vi "go striaght.vi"(7 "距离":i32, 8 "error in (no error)":errorcluster, 11 "KNR in":T1) -> (0 "error out":errorcluster, 3 "KNR out":T1)   [LabVIEW 2013]
uses:
  <userlib>/KNR OS 3.0 LabVIEW Toolkit/Type Definition/KNR3 Reference.ctl
  <userlib>/_FPGA Interface Advanced Tools/FPGA Interface Base/FPGA Interface Base.lvclass
  <userlib>/KNR OS 3.0 LabVIEW Toolkit/Type Definition/Resource.ctl
  Global 1.vi
panel:
  out "右轮位置":i32
  out "右轮初始位置":i32
  out "右轮移动了":i32
  in  "STOP":bool
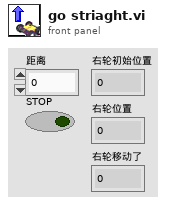
[diagram p1: front panel]
types:
  T1 = typedef "KNR3 Reference.ctl" = cluster{"FPGA Session":refnum<class "FPGA Interface Base.lvclass">, "Resource":T2}
  T2 = typedef "Resource.ctl" = enum16{"KNRm_DDRC", "KNRm_DDDD", "KNRm_DDDR", "KNRm_DDDC", "KNR"}
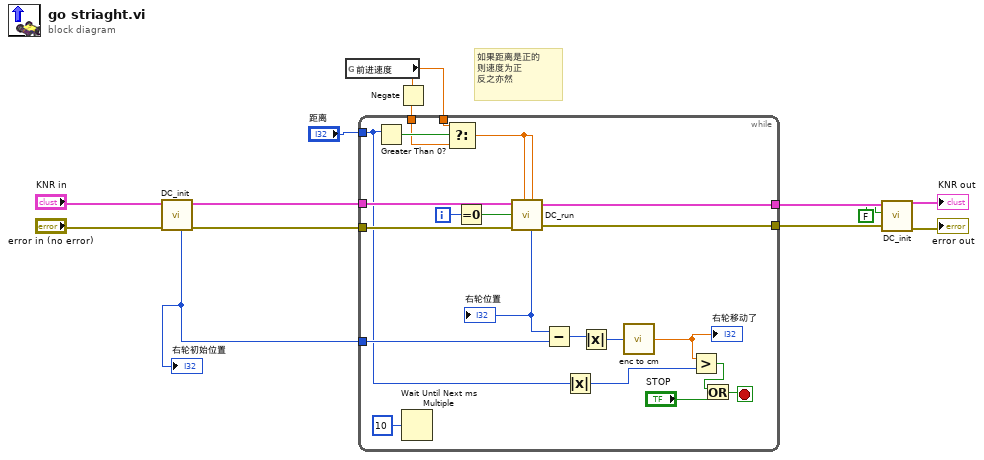
[diagram p0: block diagram]
diagram:
  # "如果距离是正的\n则速度为正\n反之亦然"
  n1 = call "DC_init.vi"("error in (no error)"="error in (no error)", "KNR in"="KNR in") -> ("error out"=w10:errorcluster, "KNR out"=w11:T1, "output\nposition 2"=w4:i32)  [unwired: 6 in, 1 out]
  "右轮初始位置" <- w4
  n2 = global read "Global 1.vi" "前进速度"() -> (w1:dbl)
  n3 = Negate(x=w1) -> (-x=w2:dbl)
  n4 = while {
    tunnel: w11 -> [w32]
    tunnel: w10 -> [w31]
    tunnel: [w23] -> w9
    tunnel: [w22] -> w8
    tunnel: w4 -> [w19]
    tunnel: "距离" -> [w18]
    tunnel: w1 -> [w17]
    tunnel: w2 -> [w16]
    i -> [w28]
    stop <- w14 stop-if-true
    n5 = Greater Than 0?(x=w18) -> (x > 0?=w33:bool)
    n6 = Wait Until Next ms Multiple(millisecond multiple=u32 10) -> ()  [unwired: 1 out]
    n7 = Select(t=w17, s=w33, f=w16) -> (s? t:f=w30:dbl)
    n8 = Equal To 0?(x=w28) -> (x = 0?=w29:bool)
    n9 = call "DC_run.vi"("KNR in"=w32, "speed_1"=w30, "reinitialize? (F)"=w29, "error in (no error)"=w31, "speed_2"=w30) -> ("KNR out"=w23:T1, "Position_2"=w20:i32, "error out"=w22:errorcluster)  [unwired: 1 in, 1 out]
    "右轮位置" <- w20
    n10 = Subtract(x=w20, y=w19) -> (x-y=w27:i32)
    n11 = Absolute Value(x=w18) -> (abs(x)=w26:i32)
    n12 = Absolute Value(x=w27) -> (abs(x)=w24:i32)
    n13 = call "enc to cm.vi"("E"=w24) -> ("CM"=w21:dbl)  [unwired: 1 in]
    "右轮移动了" <- w21
    n14 = Greater?(x=w21, y=w26) -> (0:w25:bool)
    n15 = Or(x=w25, y="STOP") -> (x .or. y?=w14:bool)
  }
  n16 = call "DC_init.vi"("error in (no error)"=w8, "Enable Motor(T)"=FALSE, "KNR in"=w9) -> ("error out"=→"error out":errorcluster, "KNR out"=→"KNR out":T1)  [unwired: 5 in, 2 out]
